vi "execute_function.vi"(6 "timeout (25000ms)":i32=25000, 8 "error in (no error)":errorcluster, 9 "data":u8[](array[numeric]), 10 "function name":string, 11 "daemon reference in":refnum<k5>) -> (0 "error out":errorcluster, 2 "response":string, 3 "daemon reference out":refnum<k5>, 5 "command out":string="random")   [LabVIEW 2017]
doc: "<b>Command: </b>\"execute_function\"\n\n<b>Description: </b>Executes a named function on the target. Make sure to provide the correct parameter byte array to provide inputs to the function.\n\n<b>Parameters: </b> \n\n 1. Name of function to run\n 2. Byte array representing parameters\ns\n<b>Note: </b>This command will only work on DEV builds of the target and as long as the relevant firmware json file has been loaded using \"load_firmware_json\" command.\n____________________________________________\nDIPC 692 Daemon API 10.0.0.1\nSam Tee - Dyson Technology Ltd\nCopyright (c) 2024, Dyson Technology Ltd"
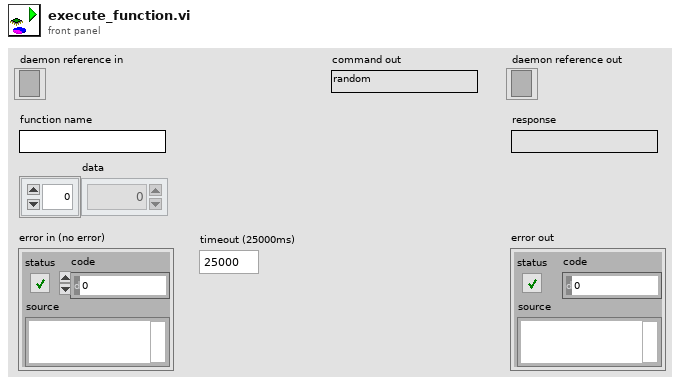
[diagram p1: front panel]
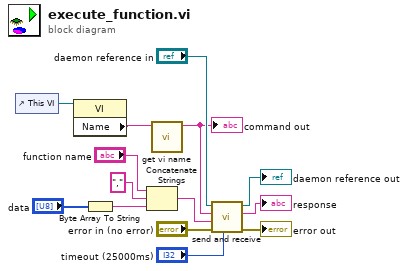
[diagram p0: block diagram]
diagram:
  n1 = control-ref of="This VI"() -> (w8:refnum<vi>)
  n2 = property class="VI"(reference=w8) -> ("Name"=w6:string)  [unwired: 1 in, 2 out]
  n3 = Byte Array To String(unsigned byte array="data") -> (string=w1:string)
  n4 = Concatenate Strings("function name", "," ("string"), w1) -> (w4:string)
  n5 = call "get vi name.vi"("library.lvlib:name.vi"=w6) -> ("vi name"=w5:string)  [unwired: 10 in]
  "command out" <- w5
  n6 = call "send and receive.vi"("timeout (25000ms)"="timeout (25000ms)", "error in (no error)"="error in (no error)", "data"=w4, "command"=w5, "daemon reference in"="daemon reference in") -> ("error out"=→"error out":errorcluster, "response"=→"response":string, "daemon reference out"=→"daemon reference out":refnum<k5>)  [unwired: 4 in]
